vi "Stop.vi"(7 "Emergency Stop? (F)":bool, 8 "error in (no error)":errorcluster, 9 "Wait for Actor Stop Timeout ms (-1)":i32=-1, 11 "API-Reference in":refnum<data-value>) -> (0 "error out":errorcluster, 1 "Timeout":bool, 2 "Final State":refnum<class "Actor.lvclass">)   [LabVIEW 2018, in "Scripting.lvlib" / "Actor.lvclass"]
uses:
  Actor.lvclass
  API-Data.ctl
  Front-Panel State.ctl
  Did Stop.ctl
  All-Enqueuers.ctl
  Broadcast Enqueuers.ctl
  Did Initialize.ctl
  Request-Enqueuers.ctl
  Get State.ctl
  State.ctl
  Stop.ctl
  <vilib>/event_ctls.llb/usereventprio.ctl
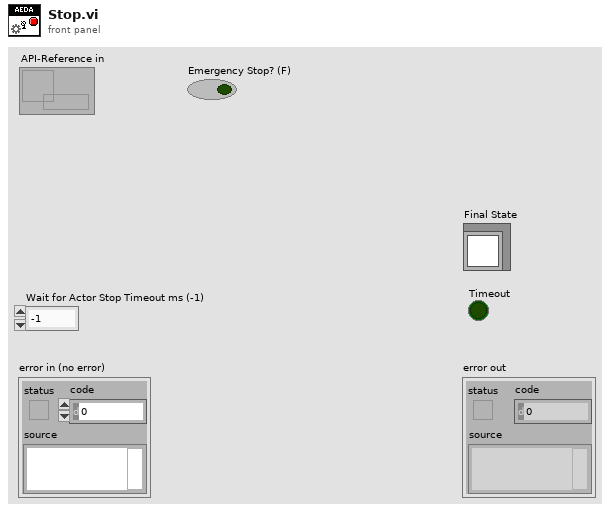
[diagram p1: front panel]
types:
  T1 = typedef "Scripting.lvlib/Actor.lvclass/API-Data.ctl" = cluster{"Launch":refnum<notifier>, "Did Stop Message":refnum<event-registration>, "Did Stop Enqueuer":refnum<user-event>, "Enqueuers":T2}
  T2 = typedef "Scripting.lvlib/Actor.lvclass/All-Enqueuers.ctl" = cluster{"Broadcasts":T3, "Requests":T4}
  T3 = typedef "Scripting.lvlib/Actor.lvclass/Broadcast Enqueuers.ctl" = cluster{"Did Initialize":refnum<user-event>}
  T4 = typedef "Scripting.lvlib/Actor.lvclass/Request-Enqueuers.ctl" = cluster{"Get State":refnum<user-event>, "Stop":refnum<user-event>}
  T5 = typedef "Scripting.lvlib/Actor.lvclass/Stop.ctl" = cluster{"Type":enum16{"Normal", "Emergency"}}
  T6 = typedef "usereventprio.ctl" = enum32{"high priority", "normal priority"}
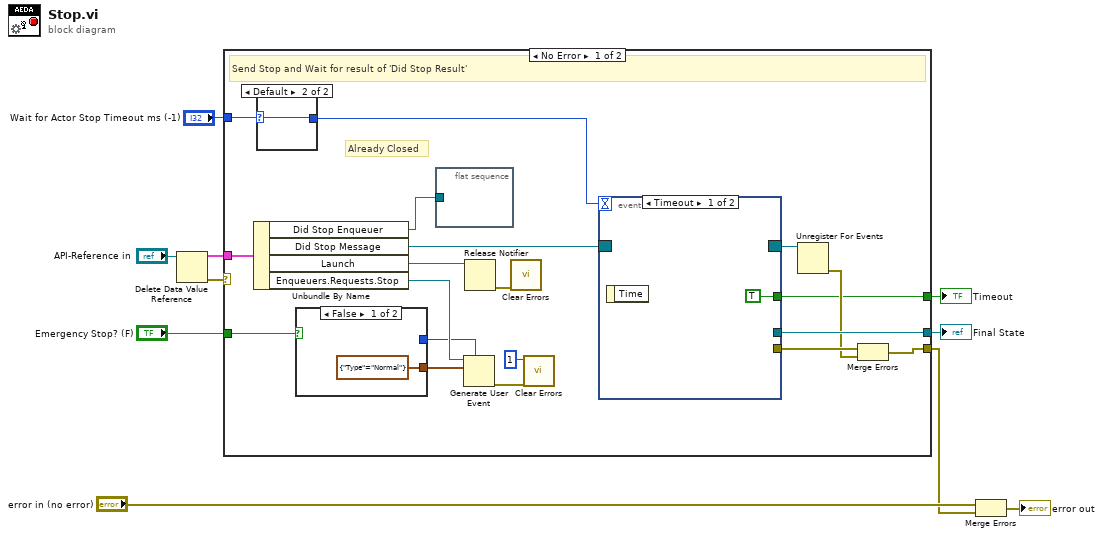
[diagram p0: block diagram]
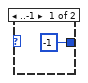
[diagram p2: hidden frame]
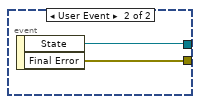
[diagram p3: hidden frame]
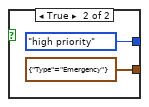
[diagram p4: hidden frame]
diagram:
  n1 = Delete Data Value Reference(data value reference="API-Reference in") -> (data value=w8:T1, error out=w7:errorcluster)  [unwired: 1 in]
  n2 = case shown="No Error" w7 {
    selector: w7 -> [_ w38]
    tunnel: w8 -> [w29 _]
    tunnel: [w19 w38] -> w3
    tunnel: "Emergency Stop? (F)" -> [w28 _]
    tunnel: "Wait for Actor Stop Timeout ms (-1)" -> [w12 _]
    tunnel: [w21 _] -> w5
    tunnel: [w17 _] -> w1
    frame No Error {
      # "Already Closed"
      # "Send Stop and Wait for result of 'Did Stop Result'"
      n3 = Unbundle By Name(w29) -> ("Did Stop Enqueuer"=w16:refnum<user-event>, "Did Stop Message"=w23:refnum<event-registration>, "Launch"=w24:refnum<notifier>, "Enqueuers.Requests.Stop"=w27:refnum<user-event>)
      n4 = case shown="Default" w12 {
        selector: w12 -> [_ w31]
        tunnel: [-1 ("Wait for \"Did Stop Broadcast\" Timeout ms (-1)") w31] -> w11
        frame ..-1 {
        }
        frame Default {
        }
      }
      n5 = case shown="False" w28 {
        tunnel: [T5 {"Type"=enum."Normal"} ("Stop") T5 {"Type"=enum."Emergency"} ("Stop")] -> w26
        tunnel: [_ usereventprio."high priority" ("priority (normal)")] -> w25
        frame False {
        }
        frame True {
        }
      }
      n6 = flat-sequence {
        tunnel: w16 -> [_]
        frame #0 {
        }
      }
      n7 = Generate User Event(priority (normal)=w25, user event=w27, event data cluster=w26) -> (error out=w14:errorcluster)  [unwired: 1 in, 1 out]
      n8 = Release Notifier(notifier=w24) -> (error out=w15:errorcluster)  [unwired: 2 in, 2 out]
      n9 = call <vilib>:"Clear Errors.vi"("error in (no error)"=w15) -> ()  [unwired: 5 in, 2 out]
      n10 = call <vilib>:"Clear Errors.vi"("error in (no error)"=w14, "specific error code to clear (0: all)"=1) -> ()  [unwired: 4 in, 2 out]
      n11 = event shown="[0] Timeout" {
        selector: w23 -> [_ _]
        dyn-events: [_ _] -> w22
        timeout: w11 -> [_ _]
        tunnel: [_ w34] -> w21
        tunnel: [_ w33] -> w20
        tunnel: [TRUE _] -> w17
        event Timeout {
          n12 = event-data() -> ()  [unwired: 1 in, 1 out]
        }
        event User Event {
          n13 = event-data() -> ("State"=w34:refnum<class "Actor.lvclass">, "Final Error"=w33:errorcluster)  [unwired: 1 in]
        }
      }
      n14 = Unregister For Events(event registration refnum=w22) -> (error out=w18:errorcluster)  [unwired: 1 in]
      n15 = Merge Errors(w20, w18) -> (w19:errorcluster)
    }
    frame Error {
      # "Stop has already been sent!"
    }
  }
  "Final State" <- w5
  "Timeout" <- w1
  n16 = Merge Errors("error in (no error)", w3) -> (→"error out":errorcluster)
